vi "Configure System.vi"   [LabVIEW 2016, in "Agilent E4980.lvlib"]
doc: "Configures the system functions of the instrument."
uses:
  <instrlib>/Agilent E4980/Agilent E4980.lvlib
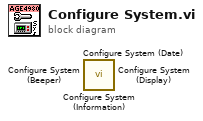
[diagram p0: block diagram]
diagram:
  n1 = call <instrlib>:"Configure System (Information).vi"() -> ()  [unwired: 10 in, 2 out]
  n2 = call <instrlib>:"Configure System (Date).vi"() -> ()  [unwired: 10 in, 2 out]
  n3 = call <instrlib>:"Configure System (Beeper).vi"() -> ()  [unwired: 10 in, 2 out]
  n4 = call <instrlib>:"Configure System (Display).vi"() -> ()  [unwired: 10 in, 2 out]
